vi "Find Center.vi"(7 "Tray Number":dbl format="%#_13g", 9 "XYZTheta":dbl[](array[numeric]), 11 "Gantry 2":refnum<k24>) -> (1 "XYZTheta Centers":dbl[][](array[numeric]), 3 "Gantry 3":refnum<k24>)   [LabVIEW 2020, in "Assembly Tray.lvclass"]
uses:
  Assembly Tray.lvclass
  Find Tray.ctl
  C:/Program Files (x86)/Aerotech/A3200/LabVIEW/2010/Bin/Aerotech.A3200.dll
  Program Files (x86)/Aerotech/A3200/LabVIEW/2010/Bin/Aerotech.A3200.dll
  Controller/Camera/Edmund Optics/Edmund Optics.lvclass
  C:/Users/hep/Documents/CMU gantry/Classes/Controller/Camera/Camera.lvclass
  Controller/Camera/Machine Vision.ctl
  Controller/Camera/Camera.lvclass
  Controller/Motion/Motion.lvclass
  Controller/Motion/A3200/A3200.lvclass
panel:
  out "Left Fiducial":dbl[](array[numeric]) format="%#.6g"
  out "Right Fiducial":dbl[](array[numeric]) format="%#.6g"
  out "Gantry":dbl[](array[numeric])
  out "Sum":dbl[](array[numeric])
  out "Camera":dbl[](array[numeric])
  in  "Carrier Tray":T1
  out "Image":T2(plugin-control)
  out "Center":dbl[](array[numeric]) format="%#.6g"
  in  "Position Number":i16
  in  "Go to Center":bool
  in  "Calculate":bool
  in  "Record Bottom":bool
  in  "Record Top":bool
  in  "Go to Bottom  Fiducial":bool
  in  "Go to Top Fiducial":bool
  in  "Joystick":bool
  in  "Stop":bool
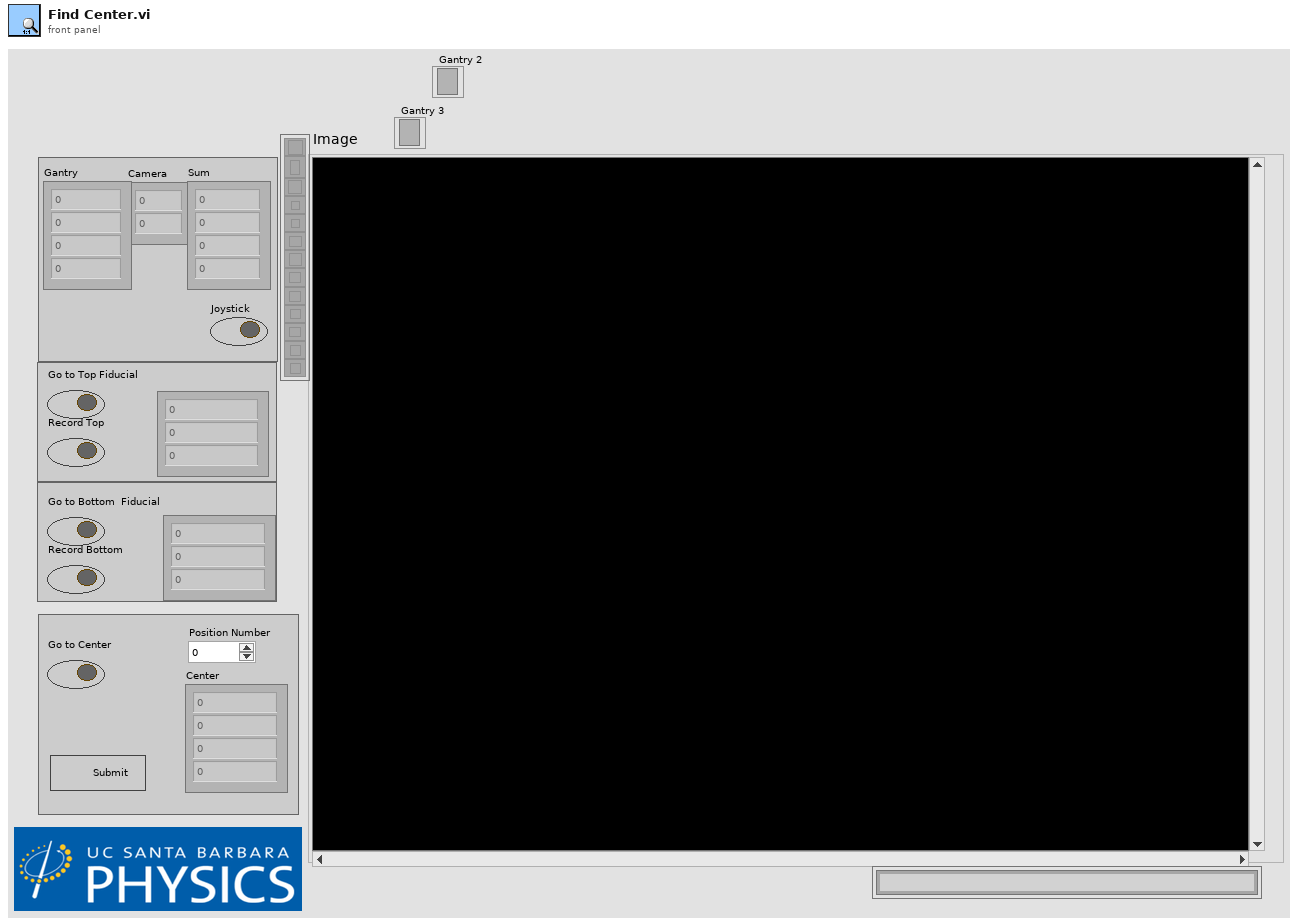
[diagram p1: front panel]
types:
  T1 = typedef "Assembly Tray.lvclass/Find Tray.ctl" = cluster{"Gantry Fiducials":dbl[], "Relative Coordinates":dbl[][], "Camera Fiducials":dbl[][], "XYZTheta Centers":dbl[][], "Workspace Center":dbl[], "Syringe Relative Coordinates":dbl[], "Gantry Region":dbl, "Fiducials":path}
  T2 = typedef "IMAQ Image.ctl" = refnum<image>
  T3 = typedef "Camera.lvclass/Machine Vision.ctl" = enum16{"None", "Tray Fiducials", "HPK Silicon", "Hexaboard", "Corner (TL, BR)", "Corner (BL, TR)"}
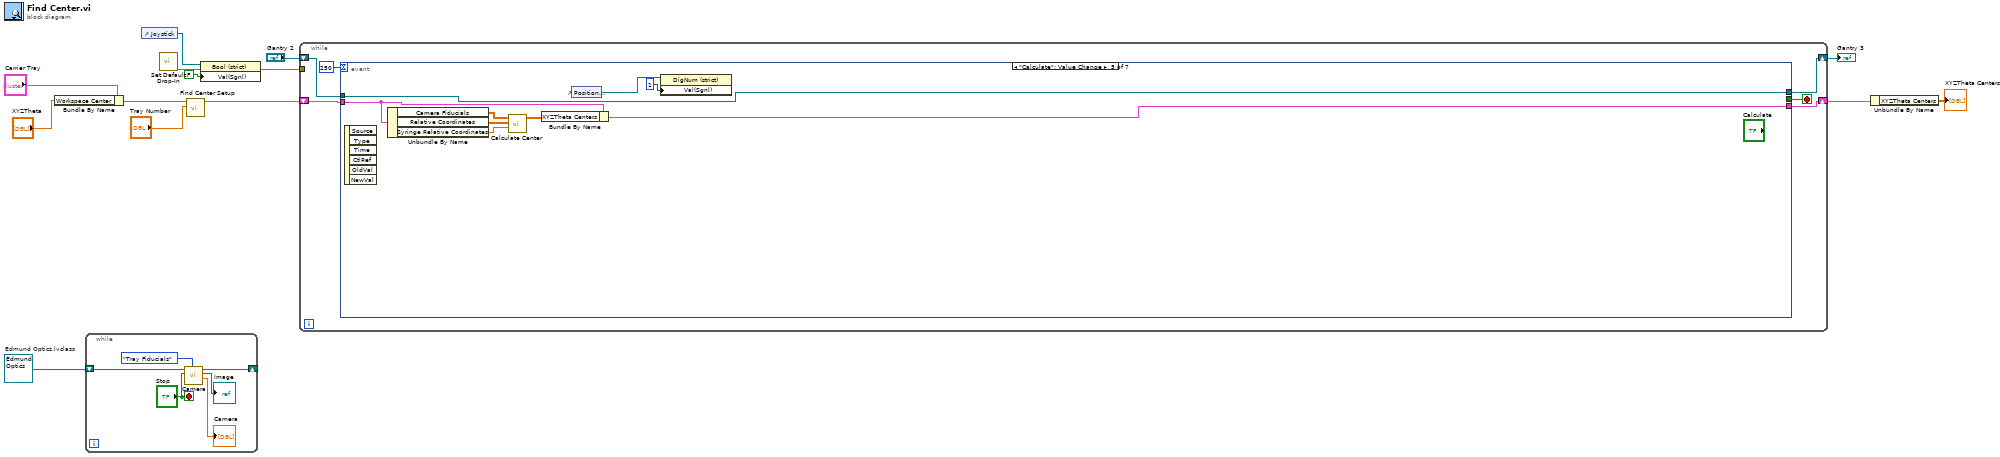
[diagram p0: block diagram]
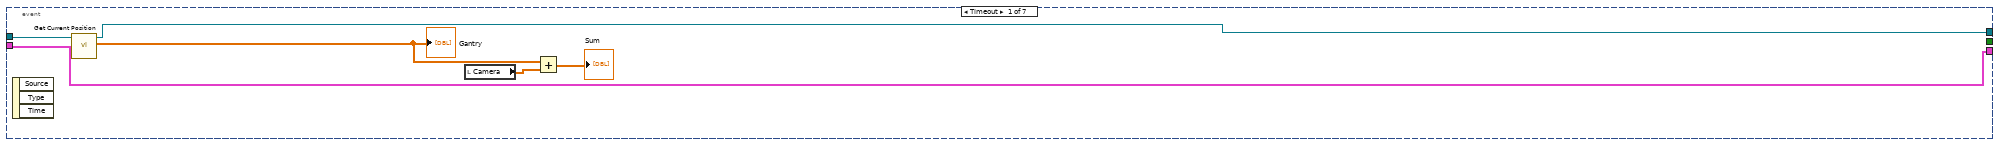
[diagram p2: hidden frame]
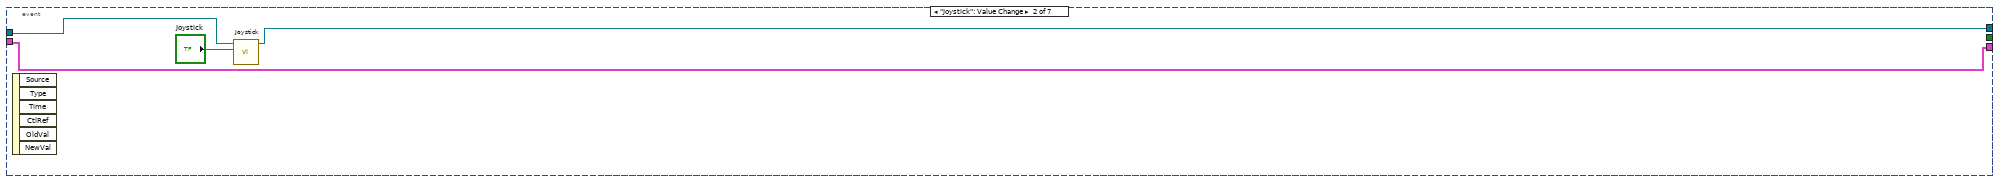
[diagram p3: hidden frame]
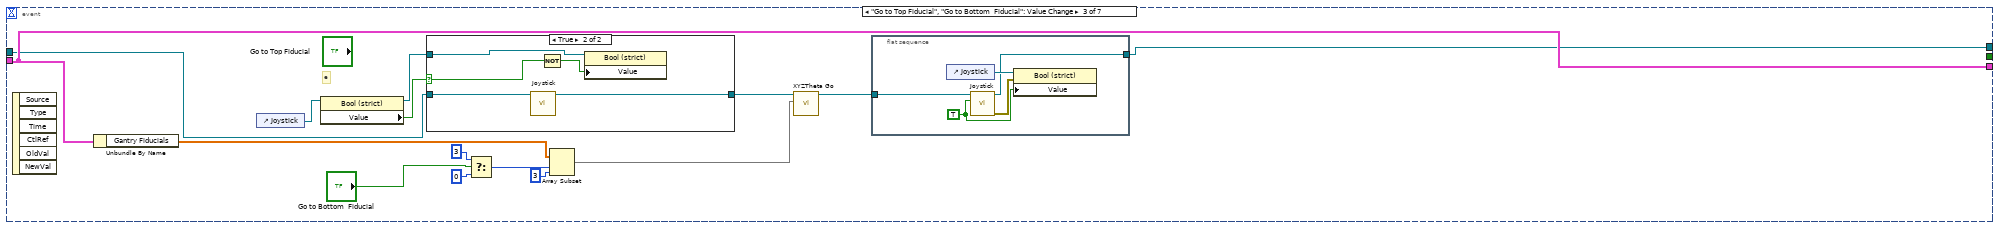
[diagram p4: hidden frame]
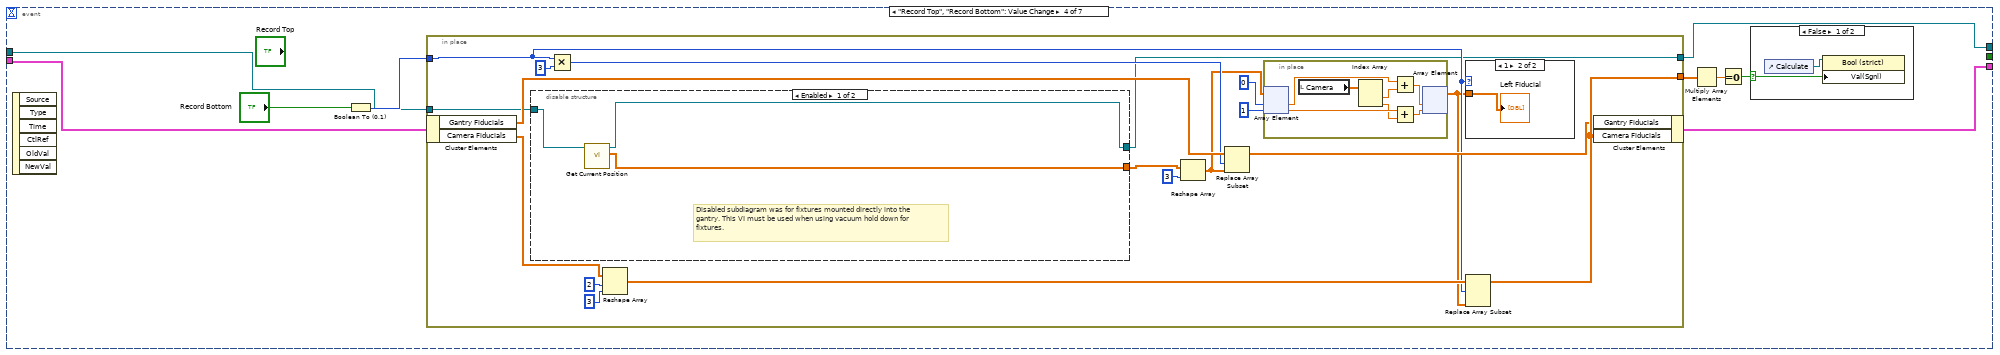
[diagram p6: hidden frame]
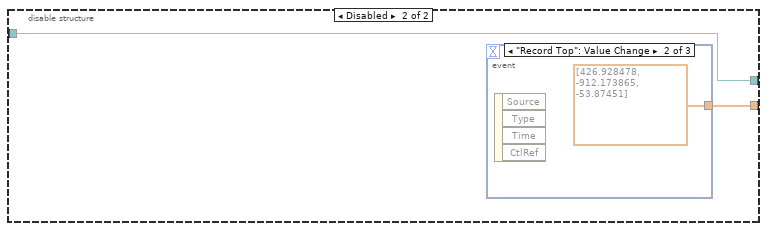
[diagram p8: hidden frame]
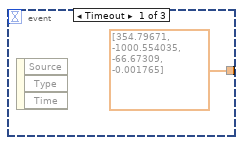
[diagram p9: hidden frame]
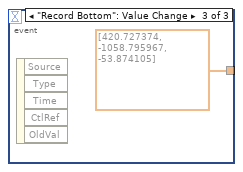
[diagram p10: hidden frame]
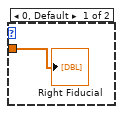
[diagram p11: hidden frame]
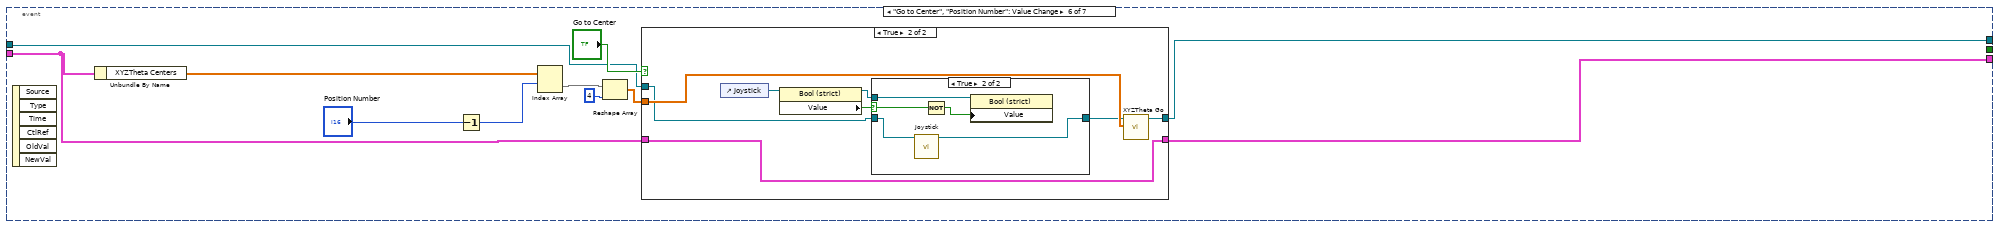
[diagram p12: hidden frame]
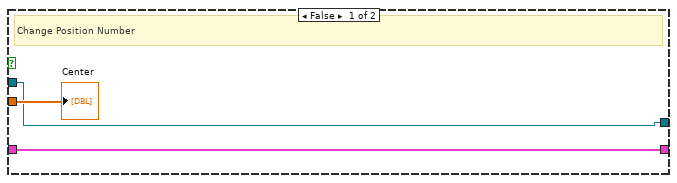
[diagram p13: hidden frame]
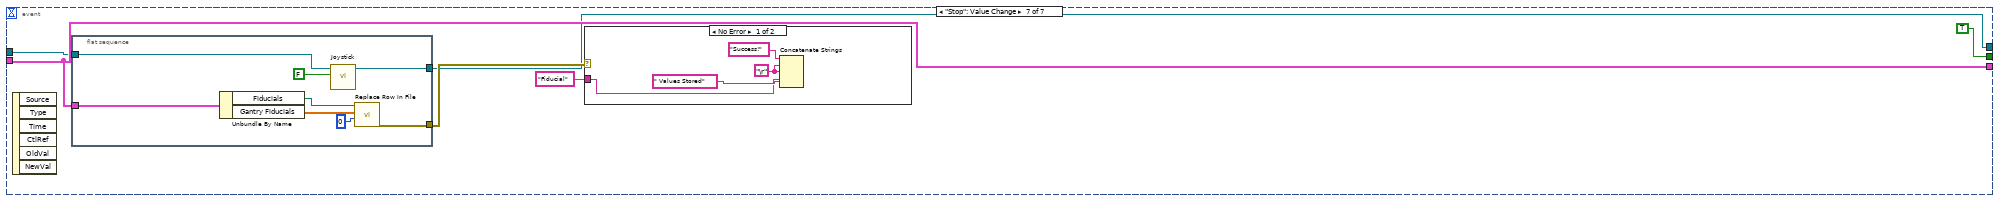
[diagram p15: hidden frame]
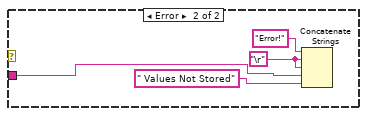
[diagram p16: hidden frame]
diagram:
  w2 = refnum<class "Edmund Optics.lvclass"> refnum  # Edmund Optics.lvclass
  n1 = Bundle By Name(cluster="Carrier Tray", "Workspace Center"="XYZTheta") -> (w8:T1)
  n2 = while {
    shift-right: [w16] -> _
    shift-left: w2 -> [w20]
    stop <- "Stop" stop-if-true
    n3 = call "Camera.vi"("Machine Vision"=Machine_Vision."Tray Fiducials", "Stop"="Stop", "Camera in"=w20) -> ("Camera"=→"Camera":dbl[], "Image"=→"Image":T2, "Camera out"=w16:refnum<class "Edmund Optics.lvclass">)  [unwired: 5 in, 1 out]
  }
  n4 = control-ref of="Joystick"() -> (w14:refnum<vi>)
  n5 = call "Set Default Drop-In.vi"() -> ("error out"=w6:errorcluster)  [unwired: 11 in]
  n6 = call "Find Center Setup.vi"("Carrier Tray"=w8, "Tray Number"="Tray Number") -> ("Assembly Tray Out"=w11:T1)  [unwired: 8 in]
  n7 = property class="Bool (strict)"(reference=w14, error in=w6, "Val(Sgnl)"=FALSE) -> (error out=w12:errorcluster)  [unwired: 1 out]
  n8 = while {
    shift-right: [w25] -> w10
    shift-left: w11 -> [w26]
    tunnel: w12 -> [_]
    shift-right: [w22] -> w3
    shift-left: "Gantry 2" -> [w21]
    stop <- w24 stop-if-true
    n9 = event shown="[4] \"Calculate\": Value Change" {
      selector: _ -> [_ _ _ _ _ _ _]
      dyn-events: _ -> [_ _ _ _ _ _ _]
      timeout: 250 -> [_ _ _ _ _ _ _]
      tunnel: [w30 w36 w51 w71 w111 w124 w149] -> w25
      tunnel: w26 -> [w30 w36 w51 w65 w115 w125 w149]
      tunnel: [_ _ _ _ _ _ TRUE] -> w24
      tunnel: w21 -> [w29 w35 w41 w64 w109 w122 w148]
      tunnel: [w27 w34 w37 w63 w109 w118 w146] -> w22
      event Timeout {
        n10 = event-data() -> ()  [unwired: 1 in, 3 out]
        n11 = call "Get Current Position.vi"("Gantry 2"=w29) -> ("XYZTheta Out"=w28:dbl[], "Gantry 3"=w27:refnum<k24>)  [unwired: 8 in, 1 out]
        "Gantry" <- w28
        n12 = local read "Camera"() -> (w32:dbl[])
        n13 = Add(x=w28, y=w32) -> (x+y=→"Sum":dbl[])
      }
      event "Joystick": Value Change {
        n14 = event-data() -> ()  [unwired: 1 in, 6 out]
        n15 = call "Joystick.vi"("Joystick"="Joystick", "Gantry 2"=w35) -> ("Gantry 3"=w34:refnum<k24>)  [unwired: 8 in, 1 out]
      }
      event "Go to Top Fiducial", "Go to Bottom  Fiducial": Value Change {
        # "e"
        n16 = event-data() -> ()  [unwired: 1 in, 6 out]
        n17 = Unbundle By Name(w51) -> ("Gantry Fiducials"=w49:dbl[])
        n18 = control-ref of="Joystick"() -> (w50:refnum<vi>)
        n19 = property class="Bool (strict)"(reference=w50) -> (reference out=w39:refnum<vi>, "Value"=w42:bool)  [unwired: 1 in, 1 out]
        n20 = case shown="True" w42 {
          selector: w42 -> [_ w62]
          tunnel: w41 -> [w57 w59]
          tunnel: [w57 w58] -> w40
          tunnel: w39 -> [_ w60]
          frame False {
          }
          frame True {
            n21 = call "Joystick.vi"("Gantry 2"=w59) -> ("Gantry 3"=w58:refnum<k24>)  [unwired: 9 in, 1 out]
            n22 = Not(x=w62) -> (.not. x?=w61:bool)
            n23 = property class="Bool (strict)"(reference=w60, "Value"=w61) -> ()  [unwired: 1 in, 2 out]
          }
        }
        n24 = Select(t=3, s="Go to Bottom  Fiducial", f=0) -> (s? t:f=w47:i32)
        n25 = Array Subset(array=w49, index=w47, length=3) -> (w43:dbl[])
        n26 = call "XYZTheta Go.vi"("XYZTheta In"=w43, "Gantry 2"=w40) -> ("Gantry 3"=w38:refnum<k24>)  [unwired: 7 in, 2 out]
        n27 = flat-sequence {
          tunnel: w38 -> [w56]
          tunnel: [w52] -> w37
          frame #0 {
            w54 = TRUE
            n28 = control-ref of="Joystick"() -> (w55:refnum<vi>)
            n29 = call "Joystick.vi"("Joystick"=w54, "Gantry 2"=w56) -> ("error out"=w53:errorcluster, "Gantry 3"=w52:refnum<k24>)  [unwired: 8 in]
            n30 = property class="Bool (strict)"(reference=w55, error in=w53, "Value"=w54) -> ()  [unwired: 2 out]
          }
        }
      }
      event "Record Top", "Record Bottom": Value Change {
        n31 = event-data() -> ()  [unwired: 1 in, 6 out]
        n32 = Boolean To (0,1)(Boolean="Record Bottom") -> (0, 1=w67:i16)
        n33 = in-place {
          in-place-border: [w85] -> w68
          in-place-border: w67 -> [w81]
          in-place-border: w64 -> [w76]
          in-place-border: [w75] -> w63
          n34 = in-place-cluster #1(w65) -> ("Gantry Fiducials"=w83:dbl[], "Camera Fiducials"=w89:dbl[][])
          n35 = disable-structure shown="Enabled" {
            disable-tunnel: w76 -> [w94 w95]
            disable-tunnel: [w93 w95] -> w75
            disable-tunnel: [w92 w96] -> w74
            frame Enabled {
              # "Disabled subdiagram was for fixtures mounted directly into the gantry. This VI must be used when using vacuum hold down for fixtures."
              n36 = call "Get Current Position.vi"("Gantry 2"=w94) -> ("XYZTheta Out"=w92:dbl[], "Gantry 3"=w93:refnum<k24>)  [unwired: 8 in, 1 out]
            }
            frame Disabled {
              n37 = event shown="[1] \"Record Top\": Value Change" {
                selector: _ -> [_ _ _]
                dyn-events: _ -> [_ _ _]
                timeout: _ -> [_ _ _]
                tunnel: [dbl[] [354.79671, -1000.554035, -66.67309, -0.001765] dbl[] [426.928478, -912.173865, -53.87451] dbl[] [420.727374, -1058.795967, -53.874105]] -> w96
                event Timeout {
                  n38 = event-data() -> ()  [unwired: 1 in, 3 out]
                }
                event "Record Top": Value Change {
                  n39 = event-data() -> ()  [unwired: 1 in, 4 out]
                }
                event "Record Bottom": Value Change {
                  n40 = event-data() -> ()  [unwired: 1 in, 5 out]
                }
              }
            }
          }
          n41 = Multiply(x=w81, y=i16 3) -> (x*y=w79:i16)
          n42 = Reshape Array(w89, 2 ("length"), 3 ("dimension size")) -> (w88:dbl[][])
          n43 = Reshape Array(w74, 3 ("dimension size")) -> (w78:dbl[])
          n44 = Replace Array Subset(array=w83, new element=w78, index=w79) -> (w82:dbl[])
          n45 = in-place {
            n46 = in-place-array #2(w78, 0, 1) -> (w105:dbl, w104:dbl)
            n47 = local read "Camera"() -> (w106:dbl[])
            n48 = Index Array(array=w106) -> (element #1=w101:dbl, element #2=w100:dbl)  [unwired: 2 in]
            n49 = Add(x=w105, y=w101) -> (x+y=w102:dbl)
            n50 = Add(x=w104, y=w100) -> (x+y=w103:dbl)
            n51 = in-place-array #2(w102, w103) -> (w77:dbl[])  [unwired: 2 out]
          }
          n52 = case shown="1" w81 {
            tunnel: w77 -> [w107 w108]
            frame 0, Default {
              "Right Fiducial" <- w107
            }
            frame 1 {
              "Left Fiducial" <- w108
            }
          }
          n53 = Replace Array Subset(array=w88, new element=w77, index (row)=w81) -> (w85:dbl[][])  [unwired: 1 in]
          n54 = in-place-cluster #1("Gantry Fiducials"=w82, "Camera Fiducials"=w85) -> (w71:T1)
        }
        n55 = Multiply Array Elements(1:w68) -> (0:w70:dbl)
        n56 = Equal To 0?(x=w70) -> (x = 0?=w69:bool)
        n57 = case shown="False" w69 {
          selector: w69 -> [w72 _]
          frame False {
            n58 = control-ref of="Calculate"() -> (w73:refnum<vi>)
            n59 = property class="Bool (strict)"(reference=w73, "Val(Sgnl)"=w72) -> ()  [unwired: 1 in, 2 out]
          }
          frame True {
          }
        }
      }
      event "Calculate": Value Change {
        n60 = event-data() -> ()  [unwired: 1 in, 6 out]
        n61 = Unbundle By Name(w115) -> ("Camera Fiducials"=w114:dbl[][], "Relative Coordinates"=w113:dbl[][], "Syringe Relative Coordinates"=w110:dbl[])
        n62 = call "Calculate Center.vi"("Syringe Coordinates"=w110, "Relative Coordinates"=w113, "Fiducial Measurements"=w114) -> ("XYZTheta Centers"=w112:dbl[][])  [unwired: 8 in]
        n63 = Bundle By Name(cluster=w115, "XYZTheta Centers"=w112) -> (w111:T1)
        n64 = control-ref of="Position Number"() -> (w117:refnum<vi>)
        n65 = property class="DigNum (strict)"(reference=w117, "Val(Sgnl)"=i16 1 ("Value (Signaling)")) -> ()  [unwired: 1 in, 2 out]
      }
      event "Go to Center", "Position Number": Value Change {
        n66 = event-data() -> ()  [unwired: 1 in, 6 out]
        n67 = Unbundle By Name(w125) -> ("XYZTheta Centers"=w128:dbl[][])
        n68 = Decrement(x="Position Number") -> (x-1=w126:i16)
        n69 = Index Array(array=w128, index (row)=w126) -> (element=w120:dbl[])  [unwired: 1 in]
        n70 = Reshape Array(w120, u32 4) -> (w119:dbl[])
        n71 = case shown="True" "Go to Center" {
          tunnel: w119 -> [w131 w137]
          tunnel: w125 -> [w130 w139]
          tunnel: [w130 w139] -> w124
          tunnel: w122 -> [w129 w133]
          tunnel: [w129 w138] -> w118
          frame False {
            # "Change Position Number"
            "Center" <- w131
          }
          frame True {
            n72 = control-ref of="Joystick"() -> (w136:refnum<vi>)
            n73 = property class="Bool (strict)"(reference=w136) -> (reference out=w134:refnum<vi>, "Value"=w135:bool)  [unwired: 1 in, 1 out]
            n74 = case shown="True" w135 {
              selector: w135 -> [_ w145]
              tunnel: w133 -> [w140 w142]
              tunnel: [w140 w141] -> w132
              tunnel: w134 -> [_ w143]
              frame False {
              }
              frame True {
                n75 = call "Joystick.vi"("Gantry 2"=w142) -> ("Gantry 3"=w141:refnum<k24>)  [unwired: 9 in, 1 out]
                n76 = Not(x=w145) -> (.not. x?=w144:bool)
                n77 = property class="Bool (strict)"(reference=w143, "Value"=w144) -> ()  [unwired: 1 in, 2 out]
              }
            }
            n78 = call "XYZTheta Go.vi"("XYZTheta In"=w137, "Gantry 2"=w132) -> ("Gantry 3"=w138:refnum<k24>)  [unwired: 7 in, 2 out]
          }
        }
      }
      event "Stop": Value Change {
        n79 = event-data() -> ()  [unwired: 1 in, 6 out]
        n80 = flat-sequence {
          tunnel: [w159] -> w151
          tunnel: w149 -> [w158]
          tunnel: w148 -> [w154]
          tunnel: [w152] -> w146
          frame #0 {
            n81 = Unbundle By Name(w158) -> ("Fiducials"=w156:path, "Gantry Fiducials"=w157:dbl[])
            n82 = call "Joystick.vi"("Joystick"=FALSE, "Gantry 2"=w154) -> ("Gantry 3"=w152:refnum<k24>)  [unwired: 8 in, 1 out]
            n83 = call "Replace Row In File.vi"("Index"=0, "Insert Array"=w157, "Path"=w156) -> ("error out"=w159:errorcluster)  [unwired: 8 in]
          }
        }
        n84 = case shown="No Error" w151 {
          tunnel: "Fiducial" -> [w160 w167]
          frame No Error {
            w161 = "\r"
            n85 = Concatenate Strings("Success!", w161, w161, w160, " Values Stored") -> ()  [unwired: 1 out]
          }
          frame Error {
            w164 = "\r"
            n86 = Concatenate Strings("Error!", w164, w164, w167, " Values Not Stored") -> ()  [unwired: 1 out]
          }
        }
      }
    }
  }
  "Gantry 3" <- w3
  n87 = Unbundle By Name(w10) -> ("XYZTheta Centers"=→"XYZTheta Centers":dbl[][])
